vi "Write.vi"(8 "error in (no error)":errorcluster, 9 "Timeout S (0)":dbl, 10 "Data":string, 11 "DeployResource in":refnum<class "DeployResource.lvclass">) -> (0 "error out":errorcluster, 2 "Bytes Written":i32, 3 "DeployResource out":refnum<class "DeployResource.lvclass">)   [LabVIEW 2020, in "PicoG-Core.lvlib" / "DeployResource.lvclass"]
uses:
  DeployResource.lvclass
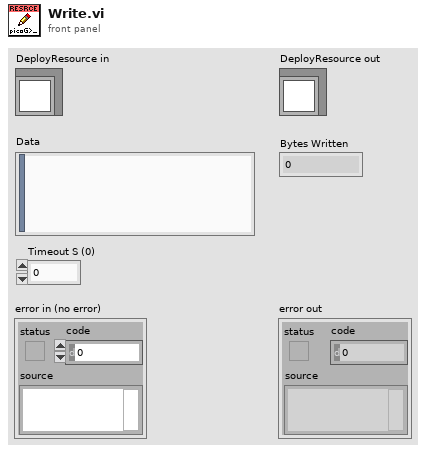
[diagram p1: front panel]
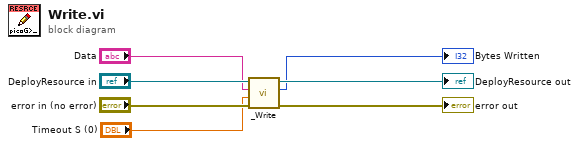
[diagram p0: block diagram]
diagram:
  n1 = call-dynamic "_Write.vi"("error in (no error)"="error in (no error)", "Timeout S (0)"="Timeout S (0)", "Data"="Data", "DeployResource in"="DeployResource in") -> ("error out"=→"error out":errorcluster, "Bytes Written"=→"Bytes Written":i32, "DeployResource out"=→"DeployResource out":refnum<class "DeployResource.lvclass">)  [unwired: 5 in]
